vi "Add Hardware Channels.vi"(8 "error in":errorcluster, 10 "channels":T1[](array[typedef]), 11 "device in":u64) -> (0 "error out":errorcluster, 3 "device out":u64)   [LabVIEW 2020, in "Communication Bus Template Scripting.lvlib"]
uses:
  Channel (Hardware Channel and Labels).ctl
  ARINC 429 Channel Definition.ctl
  Channel Parameter.ctl
  Protocol/Implementations/ARINC429/Parameter Definition.ctl
  Encoding and Decoding/Encoding.ctl
  Constants.vi
  <vilib>/NI VeriStand/Custom Device Tools/Custom Device Utility Library/NI VeriStand - Search for Item by GUID.vi
  <vilib>/NI VeriStand/Custom Device Tools/Custom Device Utility Library/NI VeriStand - Search for All Items by GUID.vi
  <vilib>/NI VeriStand/Custom Device API/NI VeriStand - Get Item Property.vi
  <vilib>/NI VeriStand/Custom Device API/Get Item Property (U16).vi
  <vilib>/NI VeriStand/Custom Device API/NI VeriStand - Get Item Children.vi
  <vilib>/NI VeriStand/Custom Device API/Get Item Property (U32).vi
  <vilib>/NI VeriStand/Custom Device API/Get Item Property (Boolean).vi
  Communication Bus Template Scripting.lvlib
  <vilib>/NI VeriStand/Custom Device Tools/Custom Device Utility Library/Custom Device Utility Library.lvlib
  <vilib>/NI VeriStand/Custom Device API/Custom Device API.lvlib
  Encoding and Decoding/Encoding and Decoding.lvlib
  Protocol/Implementations/ARINC429/ARINC 429.lvclass
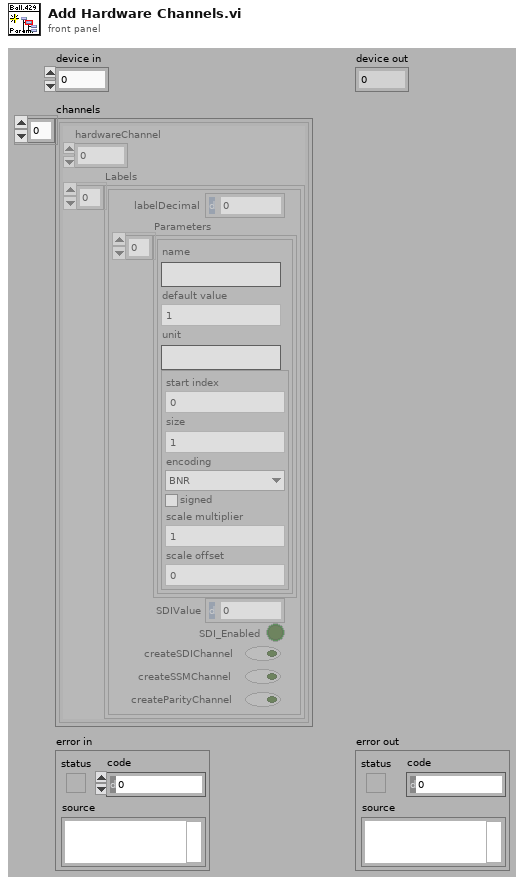
[diagram p1: front panel]
types:
  T1 = typedef "Communication Bus Template Scripting.lvlib/Channel (Hardware Channel and Labels).ctl" = cluster{"hardwareChannel":i32, "Labels":T2[]}
  T2 = typedef "Communication Bus Template Scripting.lvlib/ARINC 429 Channel Definition.ctl" = cluster{"labelDecimal":i32, "Parameters":T3[], "SDIValue":u8, "SDI_Enabled":bool, "createSDIChannel":bool, "createSSMChannel":bool, "createParityChannel":bool}
  T3 = typedef "Communication Bus Template Scripting.lvlib/Channel Parameter.ctl" = cluster{"name":string, "default value":dbl, "unit":string, "Parameter":T4}
  T4 = typedef "ARINC 429.lvclass/Parameter Definition.ctl" = cluster{"start index":i32, "size":i32, "encoding":T5, "signed":bool, "scale multiplier":dbl, "scale offset":dbl}
  T5 = typedef "Encoding and Decoding.lvlib/Encoding.ctl" = enum16{"BNR", "BCD", "Discrete"}
  T6 = typedef "Custom Device API.lvlib/Custom Device Channel Type.ctl" = enum16{"Input", "Output"}
  T7 = typedef "Custom Device API.lvlib/Custom Device Item Ref.ctl" = u64
  T8 = typedef "Custom Device API.lvlib/Custom Device Item Info.ctl" = cluster{"Name":string, "Is Channel":bool, "GUID":string, "Is Waveform":bool}
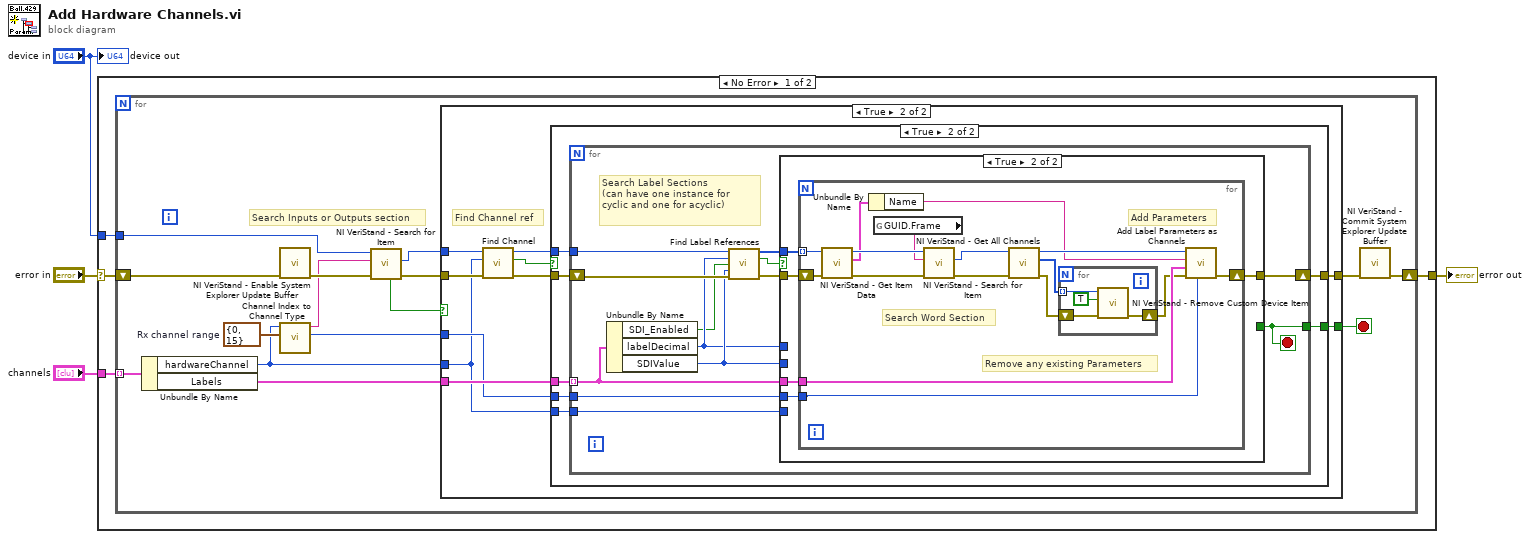
[diagram p0: block diagram]
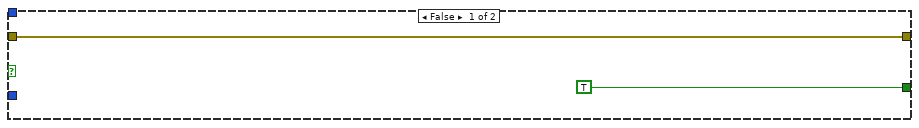
[diagram p2: hidden frame]
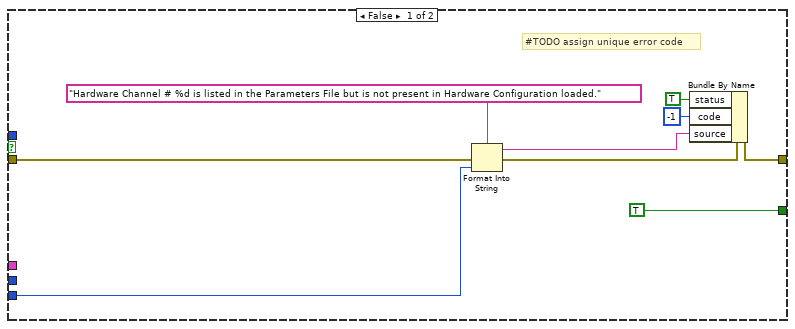
[diagram p3: hidden frame]
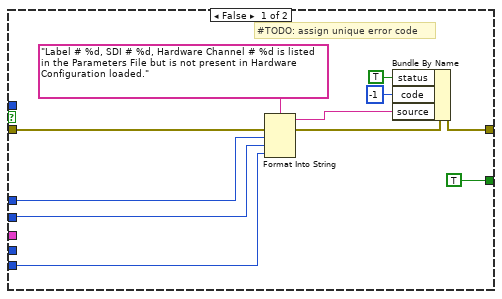
[diagram p4: hidden frame]
diagram:
  n1 = case shown="No Error" "error in" {
    selector: "error in" -> [w5 w101]
    tunnel: "channels" -> [w8 _]
    tunnel: "device in" -> [w7 _]
    tunnel: [w6 w101] -> w2
    frame No Error {
      n2 = for {
        tunnel: w7 -> [w21]
        shift-right: [w13] -> w6
        shift-left: w5 -> [w16]
        tunnel: w8 -> [w23] mode=indexing
        stop <- w17 stop-if-true
        w12 = cluster{"minimum":i32, "maximum":i32} {"minimum"=0, "maximum"=15}  # Rx channel range
        # "Search Inputs or Outputs section"
        n3 = Unbundle By Name(w23) -> ("hardwareChannel"=w11:i32, "Labels"=w22:T2[])
        n4 = call <vilib>:"NI VeriStand - Enable System Explorer Update Buffer.vi"("error in (no error)"=w16) -> ("error out"=w15:errorcluster)  [unwired: 10 in]
        n5 = call "Channel Index to Channel Type.vi"("Rx channel range"=w12, "hardware channel"=w11) -> ("custom device channel type"=w9:T6, "GUID for hardware channel type"=w10:string)  [unwired: 8 in]
        n6 = call-poly <vilib>:"NI VeriStand - Search for Item.vi"("error in"=w15, "Item GUID"=w10, "Section Ref in"=w21) -> ("error out"=w18:errorcluster, "Item Ref"=w20:T7, "Found"=w19:bool)  [unwired: 5 in, 1 out]
        n7 = case shown="True" w19 {
          tunnel: [w25 w35] -> w14
          tunnel: w22 -> [_ w32]
          tunnel: w11 -> [_ w26]
          tunnel: w20 -> [_ w28]
          tunnel: w18 -> [w25 w30]
          tunnel: [TRUE w29] -> w17
          tunnel: w9 -> [_ w27]
          frame False {
          }
          frame True {
            # "Find Channel ref"
            n8 = call "Find Channel.vi"("error in"=w30, "hardwareChannel"=w26, "item ref in"=w28) -> ("error out"=w34:errorcluster, "Found"=w33:bool, "item ref out"=w31:T7)  [unwired: 6 in]
            n9 = case shown="True" w33 {
              tunnel: [w36 w49] -> w35
              tunnel: w34 -> [w44 w51]
              tunnel: w31 -> [_ w47]
              tunnel: w32 -> [_ w50]
              tunnel: [TRUE w48] -> w29
              tunnel: w27 -> [_ w46]
              tunnel: w26 -> [w41 w45]
              frame False {
                # "#TODO assign unique error code"
                n10 = Format Into String(format string="Hardware Channel # %d is listed in the Parameters File but is not present in Hardware Configuration loaded." ("initial string"), error in=w44, w41) -> (resulting string=w38:string, error out=w37:errorcluster)  [unwired: 1 in]
                n11 = Bundle By Name(cluster=w37, "status"=TRUE, "code"=-1, "source"=w38) -> (w36:errorcluster)
              }
              frame True {
                n12 = for {
                  tunnel: w47 -> [w61]
                  tunnel: w50 -> [w63] mode=indexing
                  shift-right: [w64] -> w49
                  shift-left: w51 -> [w60]
                  tunnel: [w62] -> w48
                  tunnel: w46 -> [w53]
                  tunnel: w45 -> [w52]
                  stop <- w62 stop-if-true
                  # "Search Label Sections \n(can have one instance for cyclic and one for acyclic)"
                  n13 = Unbundle By Name(w63) -> ("SDI_Enabled"=w54:bool, "labelDecimal"=w55:i32, "SDIValue"=w56:u8)
                  n14 = call "Find Label References.vi"("item ref in"=w61, "decimalLabel"=w55, "SDI enabled"=w54, "SDI value"=w56, "error in"=w60) -> ("Array of Refs"=w58:T7[], "Found"=w57:bool, "error out"=w59:errorcluster)  [unwired: 8 in]
                  n15 = case shown="True" w57 {
                    tunnel: w59 -> [w74 w78]
                    tunnel: w58 -> [_ w77]
                    tunnel: [w65 w80] -> w64
                    tunnel: w63 -> [_ w79]
                    tunnel: w55 -> [w75 _]
                    tunnel: [TRUE _] -> w62
                    tunnel: w53 -> [_ w76]
                    tunnel: w56 -> [w71 _]
                    tunnel: w52 -> [w70 _]
                    frame False {
                      # "#TODO: assign unique error code"
                      n16 = Format Into String(format string="Label # %d, SDI # %d, Hardware Channel # %d is listed in the Parameters File but is not present in Hardware Configuration loaded.", error in=w74, w75, w71, w70) -> (resulting string=w66:string, error out=w67:errorcluster)  [unwired: 1 in]
                      n17 = Bundle By Name(cluster=w67, "status"=TRUE, "code"=-1, "source"=w66) -> (w65:errorcluster)
                    }
                    frame True {
                      n18 = for {
                        tunnel: w79 -> [w87]
                        tunnel: w77 -> [w88] mode=indexing
                        shift-right: [w83] -> w80
                        shift-left: w78 -> [w92]
                        tunnel: w76 -> [w82]
                        # "Add Parameters"
                        # "Remove any existing Parameters"
                        # "Search Word Section"
                        n19 = call <vilib>:"NI VeriStand - Get Item Data.vi"("error in (no error)"=w92, "Item Ref in"=w88) -> ("error out"=w90:errorcluster, "Item Info"=w89:T8, "Item Ref out"=w91:T7)  [unwired: 6 in, 1 out]
                        n20 = Unbundle By Name(w89) -> ("Name"=w85:string)
                        n21 = global read "Constants.vi" "GUID.Frame"() -> (w81:string)
                        n22 = call-poly <vilib>:"NI VeriStand - Search for Item.vi"("error in"=w90, "Item GUID"=w81, "Section Ref in"=w91) -> ("error out"=w95:errorcluster, "Item Ref"=w96:T7)  [unwired: 5 in, 2 out]
                        n23 = call <vilib>:"NI VeriStand - Get All Channels.vi"("error in"=w95, "Section Ref in"=w96) -> ("error out"=w93:errorcluster, "Channel Refs"=w94:T7[], "Section Ref out"=w86:T7)  [unwired: 6 in, 1 out]
                        n24 = for {
                          tunnel: w94 -> [w100] mode=indexing
                          shift-right: [w98] -> w84
                          shift-left: w93 -> [w99]
                          n25 = call <vilib>:"NI VeriStand - Remove Custom Device Item.vi"("error in (no error)"=w99, "Force Delete (F)"=TRUE, "Item Ref in"=w100) -> ("error out"=w98:errorcluster)  [unwired: 7 in, 1 out]
                        }
                        n26 = call "Add Label Parameters as Channels.vi"("channel type"=w82, "error in"=w84, "label parameters"=w87, "label name"=w85, "frame ref"=w86) -> ("error out"=w83:errorcluster)  [unwired: 5 in, 1 out]
                      }
                    }
                  }
                }
              }
            }
          }
        }
        n27 = call <vilib>:"NI VeriStand - Commit System Explorer Update Buffer.vi"("error in (no error)"=w14) -> ("error out"=w13:errorcluster)  [unwired: 10 in]
      }
    }
    frame Error {
    }
  }
  "error out" <- w2
  "device out" <- "device in"
